vi "Get Shift Data.vi"() -> (2 "Time Until Next Change":dbl, 3 "Current Shift Active?":bool)   [LabVIEW 2025]
uses:
  Globals.vi
  <vilib>/Rock Robotics/WPI/DriverStation/WPI_DriverStationAllianceInfo.ctl
panel:
  out "Shift 1 Active?":bool
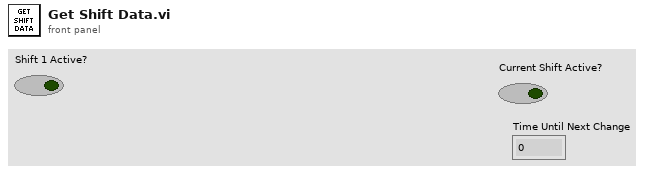
[diagram p1: front panel]
types:
  T1 = typedef "WPI_DriverStationAllianceInfo.ctl" = enum16{"Red", "Blue", "Invalid"}
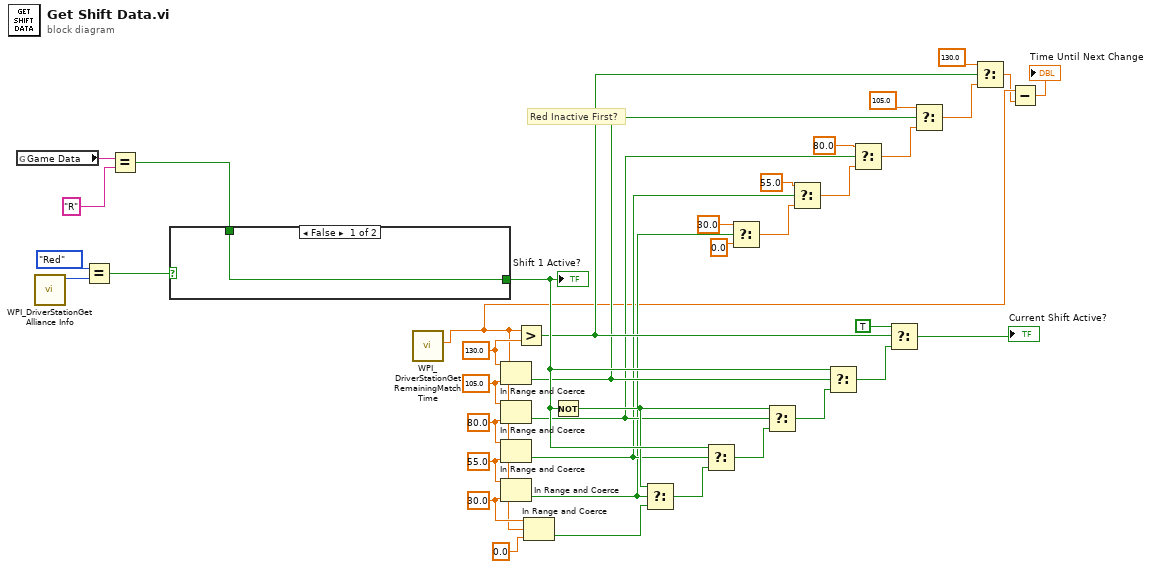
[diagram p0: block diagram]
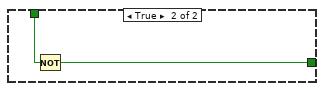
[diagram p2: hidden frame]
diagram:
  w34 = sgl 30.0 ("lower limit")
  w35 = sgl 55.0 ("lower limit")
  w36 = sgl 80.0 ("lower limit")
  w37 = sgl 105.0 ("lower limit")
  w38 = sgl 130.0 ("y")
  # "Red Inactive First?"
  n1 = global read "Globals.vi" "Game Data"() -> (w2:string)
  n2 = call <vilib>:"WPI_DriverStationGet Alliance Info.vi"() -> ("Alliance"=w5:T1)  [unwired: 6 in, 5 out]
  n3 = Equal?(x=WPI_DriverStationAllianceInfo."Red", y=w5) -> (x = y?=w3:bool)
  n4 = Equal?(x=w2, y="R") -> (x = y?=w39:bool)
  n5 = case shown="False" w3 {
    tunnel: w39 -> [w40 w42]
    tunnel: [w40 w41] -> w27
    frame False {
    }
    frame True {
      n6 = Not(x=w42) -> (.not. x?=w41:bool)
    }
  }
  "Shift 1 Active?" <- w27
  n7 = call <vilib>:"WPI_DriverStationGetRemainingMatchTime.vi"() -> ("Match Time(s)"=w8:sgl)  [unwired: 10 in, 1 out]
  n8 = In Range and Coerce(upper limit=w38, x=w8, lower limit=w37) -> (In Range?=w17:bool)  [unwired: 1 out]
  n9 = In Range and Coerce(upper limit=w37, x=w8, lower limit=w36) -> (In Range?=w15:bool)  [unwired: 1 out]
  n10 = In Range and Coerce(upper limit=w36, x=w8, lower limit=w35) -> (In Range?=w13:bool)  [unwired: 1 out]
  n11 = In Range and Coerce(upper limit=w35, x=w8, lower limit=w34) -> (In Range?=w11:bool)  [unwired: 1 out]
  n12 = Greater?(x=w8, y=w38) -> (0:w19:bool)
  n13 = In Range and Coerce(upper limit=w34, x=w8, lower limit=sgl 0.0) -> (In Range?=w24:bool)  [unwired: 1 out]
  n14 = Not(x=w27) -> (.not. x?=w25:bool)
  n15 = Select(t=w25, s=w11, f=w24) -> (s? t:f=w26:bool)
  n16 = Select(t=w27, s=w13, f=w26) -> (s? t:f=w28:bool)
  n17 = Select(t=30.0, s=w11, f=0.0) -> (s? t:f=w20:dbl)
  n18 = Select(t=w25, s=w15, f=w28) -> (s? t:f=w29:bool)
  n19 = Select(t=55.0, s=w13, f=w20) -> (s? t:f=w21:dbl)
  n20 = Select(t=w27, s=w17, f=w29) -> (s? t:f=w30:bool)
  n21 = Select(t=80.0, s=w15, f=w21) -> (s? t:f=w22:dbl)
  n22 = Select(t=TRUE, s=w19, f=w30) -> (s? t:f=→"Current Shift Active?":bool)
  n23 = Select(t=105.0, s=w17, f=w22) -> (s? t:f=w23:dbl)
  n24 = Select(t=130.0, s=w19, f=w23) -> (s? t:f=w7:dbl)
  n25 = Subtract(x=w8, y=w7) -> (x-y=→"Time Until Next Change":dbl)
